vi "Game Engine.vi"(11 "Name(\"\" to use uuid)":string="Game Engine") -> ()   [LabVIEW 2020]
uses:
  <userlib>/_NEVSTOP/Communicable State Machine(CSM)/_Support/Priority Queue/Priority Queue.lvclass/Priority Queue.ctl
  <userlib>/_NEVSTOP/Communicable State Machine(CSM)/_Polymophic/Build Register Status Message.vi
  8ce7bf74-21e7-4c02-a855-96395cb58a13.vi
  7715e510-30ac-4bfd-a476-9bbe489e10a7.vi
  48a5b973-feea-438c-9c26-a61a5607df39.vi
  <userlib>/_NEVSTOP/Communicable State Machine(CSM)/_Polymophic/Build No-Reply Asynchronous Message with Arguments.vi
  b6e4d1e1-b2b0-4aba-8ccc-cc7579037c6e.vi
  bd3d81b0-0b8a-4f04-8495-35937f111f97.vi
  f528fd67-b2af-4e3f-99d6-bbe3ff85b99e.vi
  <vilib>/numeric/Random Number (Range) U64.vi
  b905f506-a76b-4f68-b7bf-6c6363b0f74c.vi
  0e950cba-ded0-4f4e-8f3c-d05bba4cd89c.vi
  <userlib>/_NEVSTOP/Communicable State Machine(CSM)/_Support/Process/CSMP-Async Call.vi
  <userlib>/_NEVSTOP/Communicable State Machine(CSM)/_Support/GlobalEvent/GEvt-Generate Status Log.vi
  <userlib>/_NEVSTOP/Communicable State Machine(CSM)/_Support/Process/CSMP-Broadcast.vi
  <userlib>/_NEVSTOP/Communicable State Machine(CSM)/_Support/GlobalEvent/GEvt-Generate Interrupt Log.vi
  <userlib>/_NEVSTOP/Communicable State Machine(CSM)/_Support/GlobalEvent/GEvt-Generate Register Log.vi
  <userlib>/_NEVSTOP/Communicable State Machine(CSM)/_Support/Process/CSMP-Register Status.vi
  <userlib>/_NEVSTOP/Communicable State Machine(CSM)/_Support/GlobalEvent/GEvt-Generate Unregister Log.vi
  <userlib>/_NEVSTOP/Communicable State Machine(CSM)/_Support/Process/CSMP-Unregister Status.vi
  <userlib>/_NEVSTOP/Communicable State Machine(CSM)/_Support/Process/CSMP-Sync Call.vi
  <userlib>/_NEVSTOP/Communicable State Machine(CSM)/_Support/CSMQ/_CSMObj-Unlock.vi
  <userlib>/_NEVSTOP/Communicable State Machine(CSM)/_Support/Process/CSMP-PostPostMsg.vi
  <userlib>/_NEVSTOP/Communicable State Machine(CSM)/_Support/Process/CSMP-PostSendMsg.vi
  <userlib>/_NEVSTOP/Communicable State Machine(CSM)/_Support/CSMQ/_CSMObj-Lock State.vi
  <userlib>/_NEVSTOP/Communicable State Machine(CSM)/_Support/Common/Splite Reason String Part.vi
  <userlib>/_NEVSTOP/Communicable State Machine(CSM)/_Support/Common/Trim Single line Text.vi
  <userlib>/_NEVSTOP/Communicable State Machine(CSM)/_Support/CSMQ/_CSMOFGV Release.vi
  <userlib>/_NEVSTOP/Communicable State Machine(CSM)/_Support/Common/Remove Comments from Line.vi
  <userlib>/_NEVSTOP/Communicable State Machine(CSM)/_Support/Common/Splite Single-line Message.vi
  <userlib>/_NEVSTOP/Communicable State Machine(CSM)/_Support/Common/Parse Next Single-line State.vi
  <userlib>/_NEVSTOP/Communicable State Machine(CSM)/_Support/CSMQ/_CSMOFGV Dequeue.vi
  <userlib>/_NEVSTOP/Communicable State Machine(CSM)/_Support/CSMQ/_CSMObj-Log Error if in a Remote Session.vi
  <userlib>/_NEVSTOP/Communicable State Machine(CSM)/_Support/GlobalEvent/GEvt-Generate State Change Log.vi
  <userlib>/_NEVSTOP/Communicable State Machine(CSM)/_Support/GlobalEvent/GEvt-Generate Remaining States Log.vi
  <userlib>/_NEVSTOP/Communicable State Machine(CSM)/_Support/GlobalEvent/GEvt-Generate Module Destroyed Log.vi
  <userlib>/_NEVSTOP/Communicable State Machine(CSM)/_Support/GlobalEvent/GEvt-Generate Complete Log.vi
  <userlib>/_NEVSTOP/Communicable State Machine(CSM)/_Support/GlobalEvent/GEvt-Generate Module Created Log.vi
  <userlib>/_NEVSTOP/Communicable State Machine(CSM)/_Support/GlobalEvent/Cache-GEvt Filter Object.vi
  <userlib>/_NEVSTOP/Communicable State Machine(CSM)/_Support/Common/Format Timestamp.vi
  <userlib>/_NEVSTOP/Communicable State Machine(CSM)/AdvanceAPI/CSM - Revert Arguments-Safe String.vi
  <userlib>/_NEVSTOP/Communicable State Machine(CSM)/AdvanceAPI/CSM - Make String Arguments Safe.vi
  <userlib>/_NEVSTOP/Communicable State Machine(CSM)/AdvanceAPI/CSM - Break Down Multiple States String.vi
  <userlib>/_NEVSTOP/Communicable State Machine(CSM)/AdvanceAPI/CSM - Compact Multiple States.vi
  <userlib>/_NEVSTOP/Communicable State Machine(CSM)/Utility/Trim Both Whitespace.vi
  <vilib>/numeric/sub_Random U32.vi
  <userlib>/_NEVSTOP/Communicable State Machine(CSM)/_Support/CSMQ/_CSMObj-Message Check.vi
  <userlib>/_NEVSTOP/Communicable State Machine(CSM)/_Support/CSMQ/_CSMObj-Enqueue Cross-Module Message.vi
  <userlib>/_NEVSTOP/Communicable State Machine(CSM)/_Support/CSMQ/_CSMOFGV Get.vi
  <userlib>/_NEVSTOP/Communicable State Machine(CSM)/_Support/GlobalEvent/GEvt-Generate with Rule Check.vi
  <userlib>/_NEVSTOP/Communicable State Machine(CSM)/_Support/FGV-BroadcastRegistry/Cache-Broadcast Registry Search Result.vi
  <userlib>/_NEVSTOP/Communicable State Machine(CSM)/AdvanceAPI/CSM - Register Status Change.vi
  <userlib>/_NEVSTOP/Communicable State Machine(CSM)/AdvanceAPI/CSM - Unregister Status Change.vi
  <userlib>/_NEVSTOP/Communicable State Machine(CSM)/_Support/Common/Hex Str to U8 Data.vi
  <userlib>/_NEVSTOP/Communicable State Machine(CSM)/_Support/Common/Concatenate State with Arguments.vi
  <userlib>/_NEVSTOP/Communicable State Machine(CSM)/_Support/Common/U8 Data to Hex Str.vi
  <userlib>/_NEVSTOP/Communicable State Machine(CSM)/_Support/Priority Queue/Dequeue Element.vi
  <userlib>/_NEVSTOP/Communicable State Machine(CSM)/AdvanceAPI/CSM - Keywords.vi
  <userlib>/_NEVSTOP/Communicable State Machine(CSM)/_Support/Priority Queue/Enqueue Element.vi
  <userlib>/_NEVSTOP/Communicable State Machine(CSM)/_Support/GlobalEvent/LogFilter/Filter Check.vi
  <userlib>/_NEVSTOP/Communicable State Machine(CSM)/_Support/GlobalEvent/FGV-GlobalEventRef.vi
  <userlib>/_NEVSTOP/Communicable State Machine(CSM)/_Support/GlobalEvent/global-GEvnt Filter Change Flag.vi
  <userlib>/_NEVSTOP/Communicable State Machine(CSM)/FGV-GEvt Filter Obj.vi
  <userlib>/_NEVSTOP/Communicable State Machine(CSM)/_Support/CSMQ/_CSMOFGV Obtain.vi
  <userlib>/_NEVSTOP/Communicable State Machine(CSM)/_Support/GlobalEvent/LogFilter/CheckVIs/Group Check - CSM.vi
  <userlib>/_NEVSTOP/Communicable State Machine(CSM)/_Support/GlobalEvent/LogFilter/CheckVIs/Group Check - LogType.vi
  <userlib>/_NEVSTOP/Communicable State Machine(CSM)/_Support/GlobalEvent/LogFilter/CheckVIs/Group Check - State.vi
  <userlib>/_NEVSTOP/Communicable State Machine(CSM)/_Support/GlobalEvent/LogFilter/CheckVIs/CSM Check - LogType.vi
  <userlib>/_NEVSTOP/Communicable State Machine(CSM)/_Support/GlobalEvent/LogFilter/CheckVIs/CSM Check - State.vi
  <userlib>/_NEVSTOP/Communicable State Machine(CSM)/_Support/GlobalEvent/LogFilter/CheckVIs/CSM Check - StateType.vi
  <userlib>/_NEVSTOP/Communicable State Machine(CSM)/_Support/GlobalEvent/LogFilter/CheckVIs/Group Check - StateType.vi
  <userlib>/_NEVSTOP/Communicable State Machine(CSM)/_Support/CSMQ/_CSMOFGV.vi
  <userlib>/_NEVSTOP/Communicable State Machine(CSM)/_Support/Error/CSM Not Allowed Message.vi
  <userlib>/_NEVSTOP/Communicable State Machine(CSM)/_Support/GlobalEvent/FGV-StatusChangeEventRef.vi
  <userlib>/_NEVSTOP/Communicable State Machine(CSM)/_Support/FGV-BroadcastRegistry/global-CSMQ FGV Change Flag.vi
  <userlib>/_NEVSTOP/Communicable State Machine(CSM)/_Support/FGV-BroadcastRegistry/global-Broadcast Cache Change Flag.vi
  <userlib>/_NEVSTOP/Communicable State Machine(CSM)/_Support/BroadcastRegistry/HelperVI/Broadcast Item Key.vi
  <userlib>/_NEVSTOP/Communicable State Machine(CSM)/_Support/FGV-BroadcastRegistry/FGV-BroadcastRegistry.vi
  <userlib>/_NEVSTOP/Communicable State Machine(CSM)/_Support/Message/Parse Register Message.vi
  <userlib>/_NEVSTOP/Communicable State Machine(CSM)/_Support/Message/Parse Unregister Message.vi
  <userlib>/_NEVSTOP/Communicable State Machine(CSM)/addons/API-String-Arugments-Support/_Support/Convert API String Arguments to Data(variant).vi
  <userlib>/_NEVSTOP/Communicable State Machine(CSM)/addons/API-String-Arugments-Support/_Support/Data To API String Arguments.vi
  <userlib>/_NEVSTOP/Communicable State Machine(CSM)/_Support/Message/Parse State with Arguments String.vi
  <userlib>/_NEVSTOP/Communicable State Machine(CSM)/Communicable State Machine.lvlib
panel:
  out "Error Occurred":errorcluster
  out "State History":string
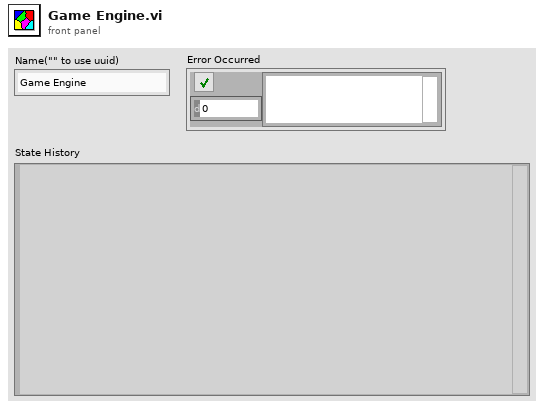
[diagram p1: front panel]
types:
  T1 = enum32{"Invalid", "Standard", "Closed", "Hidden", "Minimized", "Maximized"}
  T2 = enum32{"invalid app kind", "Development System", "Run Time System", "Student Edition", "Embedded LabVIEW", "Evaluation", "Custom"}
  T3 = typedef "Communicable State Machine.lvlib/_CSM_Response Source Message.ctl" = cluster{"‘State":string, "’Arguments":string, "’Error":errorcluster}
  T4 = cluster{"Current VI Reference":refnum<vi>, "Close Panel on Exit?":bool}
  T5 = cluster{"Core":cluster{"Current VI Reference":refnum<vi>, "Close Panel on Exit?":bool}, "Your Boolean data":bool, "current":timestamp, "timeseq":cluster{"SEQ":i32[], "time":i32}, "score":i32, "TAPSEQ":i32[], "elapsed":dbl, "load":dbl}
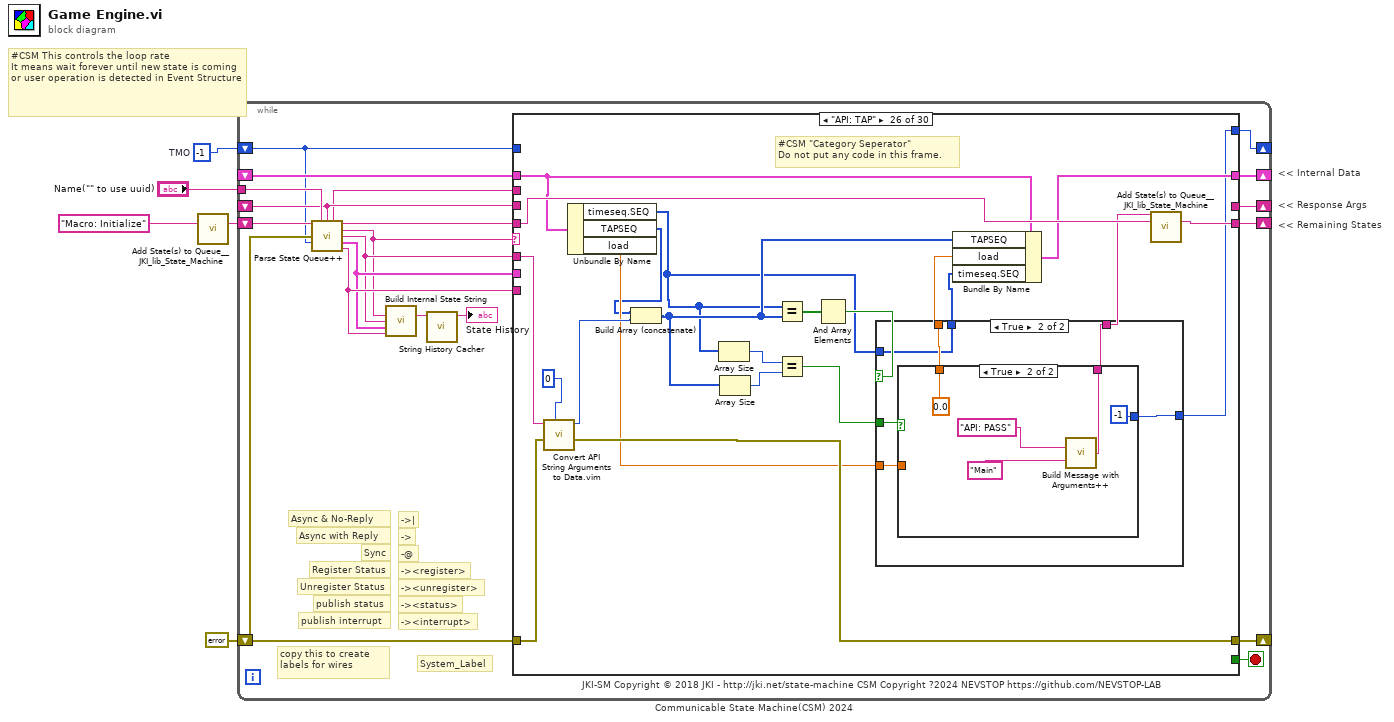
[diagram p0: block diagram]
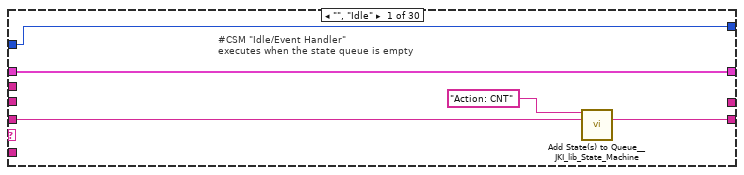
[diagram p2: hidden frame]
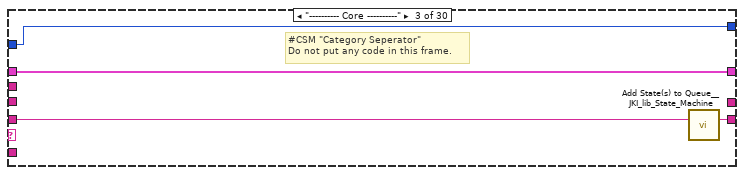
[diagram p4: hidden frame]
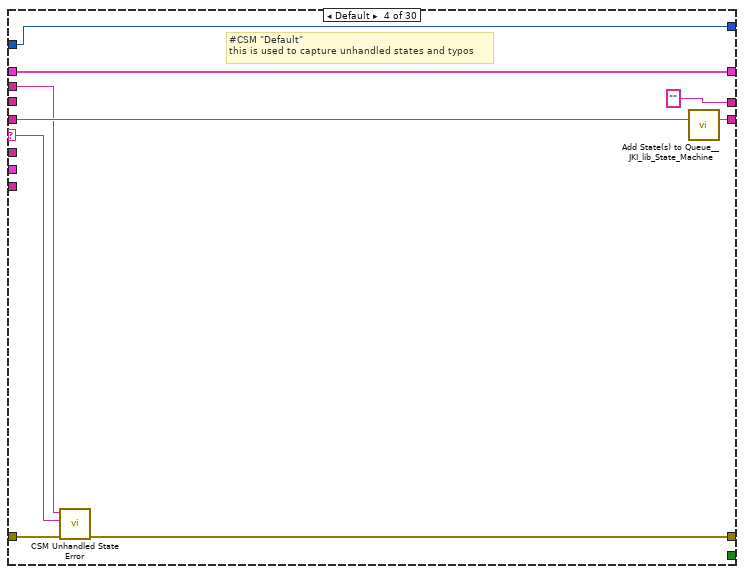
[diagram p5: hidden frame]
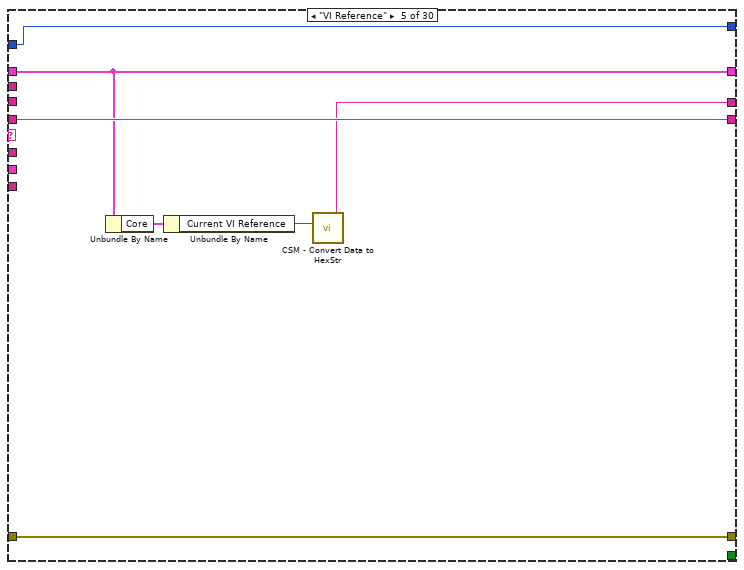
[diagram p6: hidden frame]
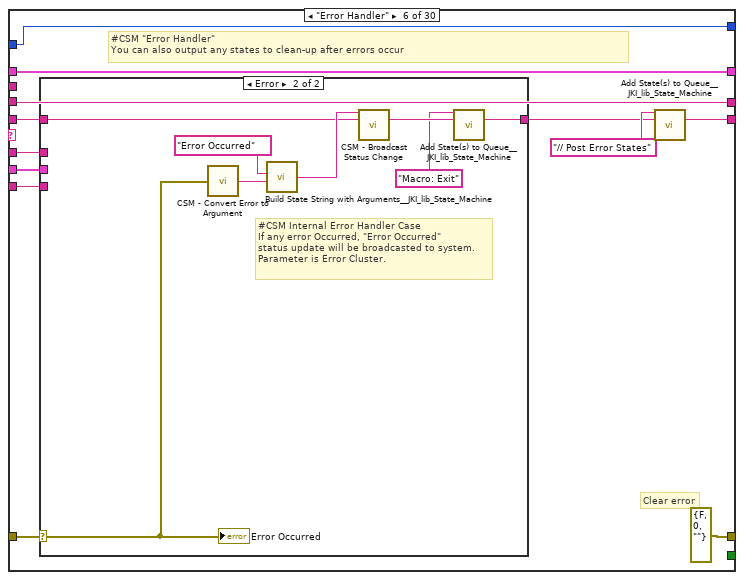
[diagram p7: hidden frame]
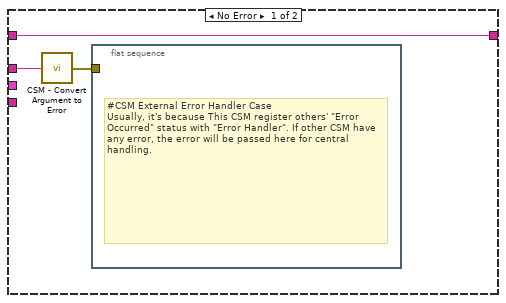
[diagram p8: hidden frame]
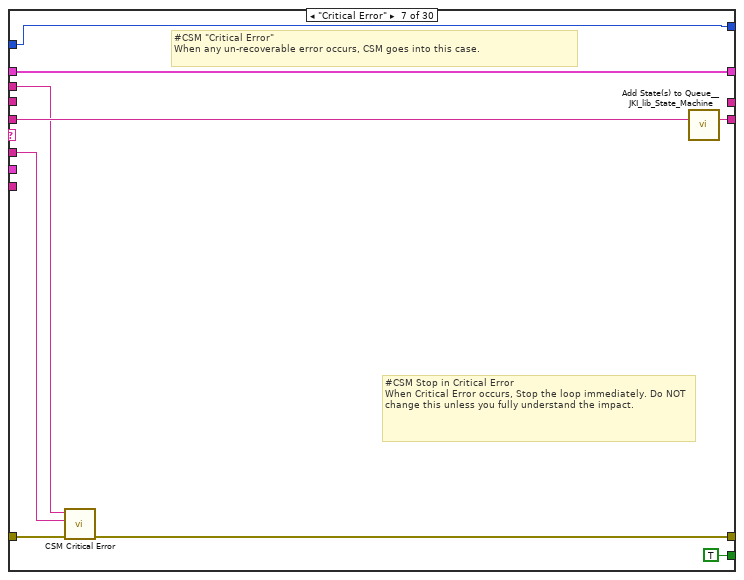
[diagram p9: hidden frame]
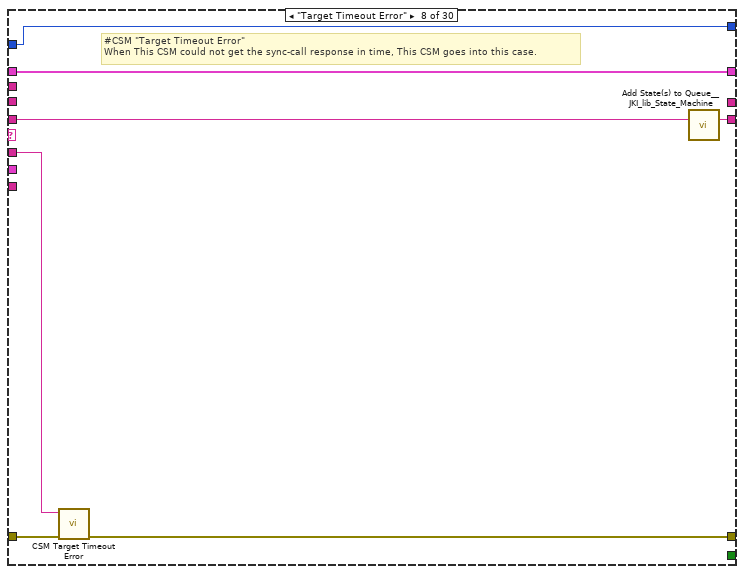
[diagram p10: hidden frame]
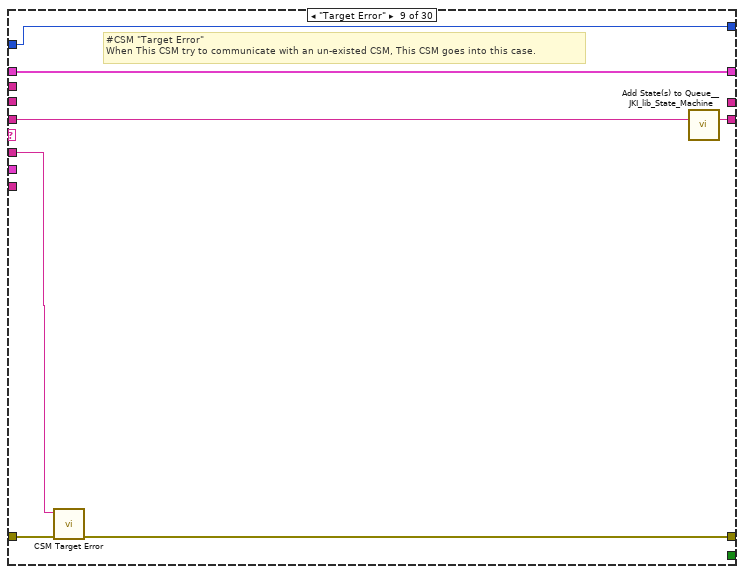
[diagram p11: hidden frame]
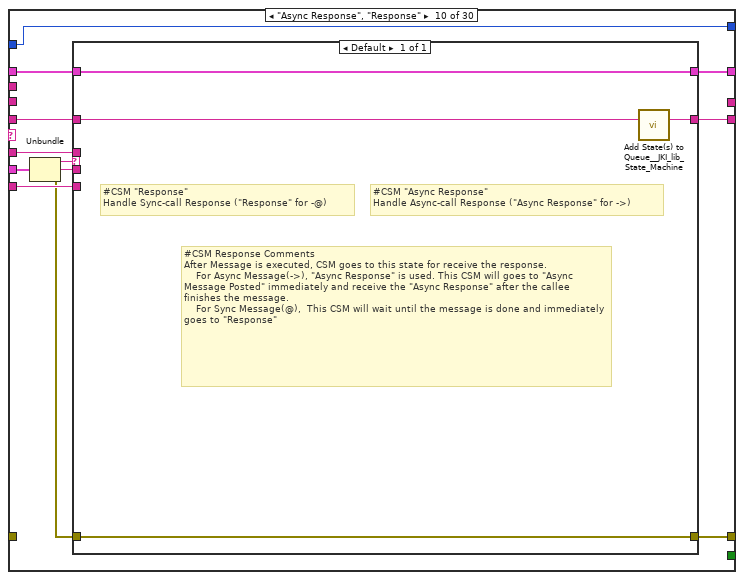
[diagram p12: hidden frame]
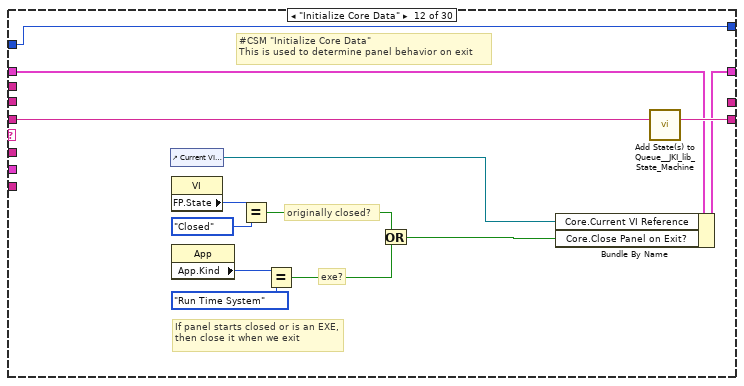
[diagram p14: hidden frame]
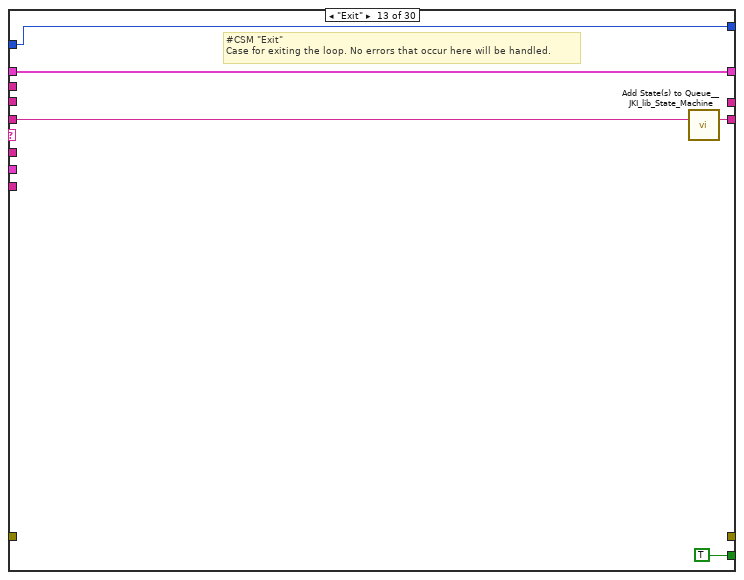
[diagram p15: hidden frame]
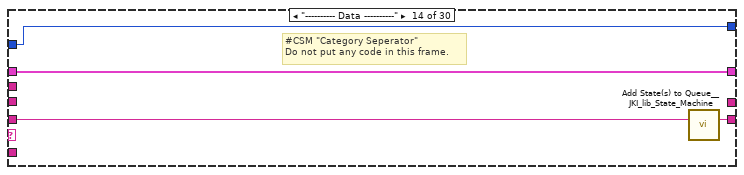
[diagram p16: hidden frame]
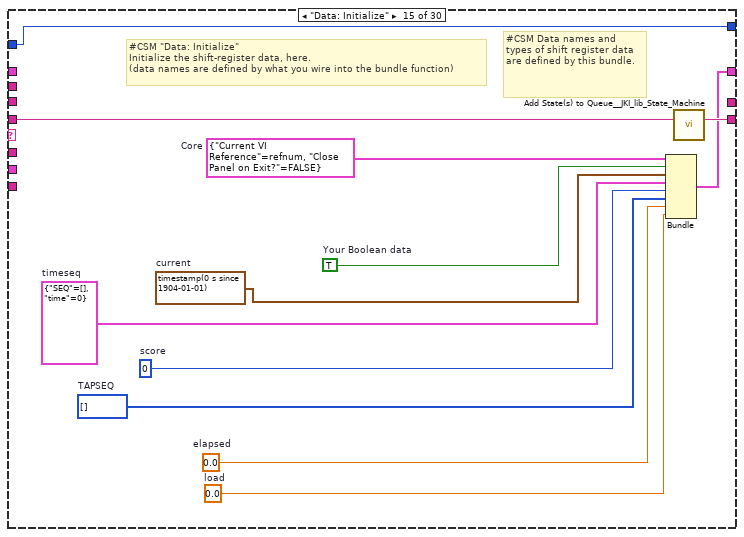
[diagram p17: hidden frame]
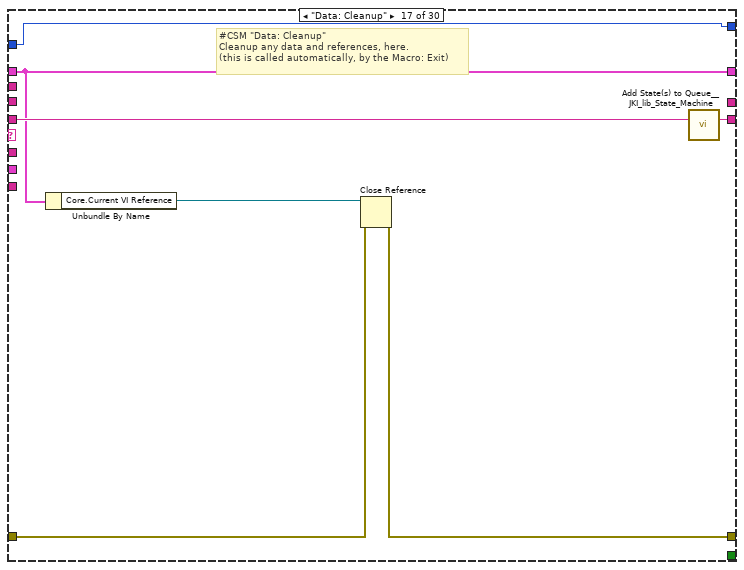
[diagram p19: hidden frame]
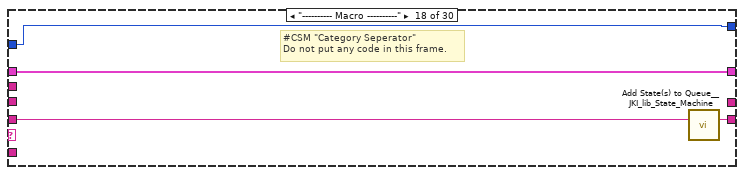
[diagram p20: hidden frame]
diagram:
  w1 = -1  # TMO
  # "#CSM This controls the loop rate\nIt means wait forever until new state is coming or user operation is detected in Event Structure"
  # "<< Internal Data"
  # "<< Response Args"
  # "<< Remaining States"
  n1 = call <vilib>:"Add State(s) to Queue__JKI_lib_State_Machine.vi"("State(s) in (\"\")"="Macro: Initialize" ("Init State(\"Macro: Initialize\")")) -> ("States Out"=w3:string)  [unwired: 14 in]
  n2 = while "Communicable State Machine(CSM) 2024" {
    shift-right: [w20] -> _
    shift-left: _ -> [w19]
    shift-right: [w23] -> _
    shift-left: errorcluster {"status"=FALSE, "code"=0, "source"=""} ("error out") -> [w8]
    shift-right: [w22] -> _
    shift-left: w3 -> [w24]
    tunnel: "Name(\"\" to use uuid)" -> [w17]
    shift-right: [w18] -> _
    shift-left: _ -> [w10]
    shift-right: [w7] -> _
    shift-left: w1 -> [w6]
    stop <- w21 stop-if-true
    # "-><interrupt>"
    # "-><status>"
    # "-><unregister>"
    # "-><register>"
    # "-@"
    # "->"
    # "->|"
    # "publish interrupt"
    # "publish status"
    # "Unregister Status"
    # "Register Status"
    # "Sync"
    # "Async with Reply"
    # "Async & No-Reply"
    # "JKI-SM Copyright © 2018 JKI - http://jki.net/state-machine CSM Copyright ?2024 NEVSTOP https://github.com/NEVSTOP-LAB"
    # "copy this to create labels for wires"
    # "System_Label"
    n3 = call <userlib>:"Parse State Queue++.vi"("State Queue"=w24, "Name(\"\" to use uuid)"=w17, "Response Arguments"=w10, "Error In (no error)"=w8, "Dequeue Timeout(0ms)"=w6) -> ("Name Used"=w9:string, "Remaining States"=w25:string, "Current State"=w11:string, "Arguments"=w12:string, ">> Response Source Message >>"=w13:T3, ">> Source CSM >>"=w14:string)  [unwired: 5 in]
    n4 = call <userlib>:"Build Internal State String.vi"("State"=w11, "Arguments (\"\")"=w12, ">> Response Source Message >>"=w13, "Source (\"\")"=w14) -> ("State with Arguments"=w15:string)  [unwired: 11 in]
    n5 = call <userlib>:"String History Cacher.vi"("String"=w15) -> ("String Cache"=→"State History":string)  [unwired: 10 in]
    n6 = case shown="\"API: TAP\"" w11 {
      selector: w11 -> [_ _ _ w42 _ _ _ _ _ _ _ _ _ _ _ _ _ _ _ _ _ _ _ _ _ _ _ _ _ _]
      tunnel: w25 -> [w28 w33 w37 w46 w52 w59 w85 w92 w99 w110 w118 w131 w136 w140 w152 w155 w162 w166 w170 w188 w191 w200 w213 w231 w249 w267 w296 w305 w333 w348]
      tunnel: w12 -> [_ _ _ _ _ w58 w81 w89 w96 w104 _ _ _ _ _ _ _ _ _ _ _ w205 w211 _ w242 w265 _ _ _ _]
      tunnel: w19 -> [w30 w32 w35 w44 w51 w64 w83 w90 w97 w108 w117 w125 w134 w138 _ w154 w157 w164 w180 w186 w190 w195 w216 w221 w238 w261 w294 w311 w322 w345]
      tunnel: [_ _ _ w39 w53 errorcluster {"status"=FALSE, "code"=0, "source"=""} ("error out") w78 w87 w94 w111 _ _ _ _ _ _ w158 _ _ _ _ w198 w208 w222 w243 w257 _ w313 w319 _] -> w23
      tunnel: w8 -> [_ _ _ w40 w53 w62 w79 w88 w95 _ _ _ _ _ _ _ w159 _ _ _ _ w204 w210 w223 w241 w263 _ w298 w320 _]
      tunnel: [w29 w33 w36 w45 w52 w60 w84 w91 w98 w109 w118 w130 w135 w139 w151 w155 w161 w165 w181 w187 w191 w201 w214 w232 w250 w268 w295 w306 w334 w347] -> w22
      tunnel: [_ _ _ _ _ _ TRUE _ _ _ _ _ TRUE _ _ _ _ _ _ _ _ _ _ _ _ _ _ _ _ _] -> w21
      tunnel: [w30 w32 w35 w44 w51 w64 w83 w90 w97 w107 w117 w129 w134 w138 w150 w154 w157 w164 w180 w186 w190 w203 w215 w220 w236 w260 w294 w312 w321 w344] -> w20
      tunnel: w14 -> [_ _ _ _ _ w57 _ _ _ w105 _ _ _ _ _ _ _ _ _ _ _ _ _ _ _ _ _ _ _ _]
      tunnel: w13 -> [_ _ _ _ _ w56 _ _ _ w106 _ _ _ _ _ _ _ _ _ _ _ _ _ _ _ _ _ _ _ _]
      tunnel: [_ _ _ "" w48 w55 _ _ _ _ _ _ _ _ _ _ _ _ _ _ _ _ _ _ _ _ _ _ _ _] -> w18
      tunnel: w9 -> [_ _ _ w41 _ _ w80 _ _ _ _ _ _ _ _ _ _ _ w167 _ _ _ _ _ _ _ _ _ _ _]
      tunnel: w10 -> [_ _ _ _ _ w55 _ _ _ _ _ _ _ _ _ _ _ _ _ _ _ _ _ _ _ _ _ _ _ _]
      tunnel: [w27 w31 w34 w38 w47 w54 w77 w86 w93 w100 w116 w119 w132 w137 w145 w153 w156 w163 w175 w182 w189 w196 w212 -1 ("TMO") 100 ("TMO") w256 w293 w297 w323 -1 ("TMO")] -> w7
      tunnel: w6 -> [w27 w31 w34 w38 w47 w54 w77 w86 w93 w100 w116 w119 w132 w137 w145 w153 w156 w163 w175 w182 w189 w196 w212 _ _ _ w293 w297 _ _]
      frame "", "Idle" {
        # "#CSM \"Idle/Event Handler\"\nexecutes when the state queue is empty"
        n7 = call <vilib>:"Add State(s) to Queue__JKI_lib_State_Machine.vi"("State(s) in Front (\"\")"="Action: CNT" ("State(s) in Front (\"\")"), "State(s) in (\"\")"=w28) -> ("States Out"=w29:string)  [unwired: 13 in]
      }
      frame "CSM Documentation" {
        # "#CSM Documentation"
        # "#CSM State Syntax\n\n// Comment line, all text to the right of “//” will be ignored\n// Local Message Example\nDoSth: DoA >> Arguments\n\n// Sync Call Example\nAPI: xxxx >> Arguments -@ TargetModule\n\n// Async Call Example\nAPI: xxxx >> Arguments -> TargetModule\n\n// Async Call without Reply Example\nAPI: xxxx >> Arguments ->| TargetModule\n\n// Broadcast normal status:\nStatus >> StatusArguments  -><status>\n\n// Broadcast Interrupt status:\nInterrupt >> StatusArguments  -><interrupt>\n\n// Register Source Module's status to Handler Module\nStatus@Source Module >> Handler Module@Handler Module -><register>\n\n// Unegister Source Module's status\nStatus@Source Module >> Handler Module -><unregister>"
        # "#CSM README FIRST\n\nCommunicable State Machine(CSM) is a LabVIEW application framework that builds upon JKI State Machine(JKISM). It follows the pattern of JKISM and extends the keywords to describe message communication between modules, including concepts such as Sync-Message, Async-Message, Subscription/Unsubscription of status - essential elements for creating reusable code modules. For more information, please visit the CSM wiki: https://nevstop-lab.github.io/CSM-Wiki/\n\nFor instructions on JKI State Machine, visit: \n    http://jki.net/state-machine/\nFor information about CSM, visit: \n    https://github.com/NEVSTOP-LAB"
        # "#CSM \"Documentation\"\nCase for holding CSM Documenation"
      }
      frame "---------- Core ----------" {
        # "#CSM \"Category Seperator\"\nDo not put any code in this frame."
        n8 = call <vilib>:"Add State(s) to Queue__JKI_lib_State_Machine.vi"("State(s) in (\"\")"=w37) -> ("States Out"=w36:string)  [unwired: 14 in]
      }
      frame Default {
        # "#CSM \"Default\"\nthis is used to capture unhandled states and typos"
        n9 = call <userlib>:"CSM Unhandled State Error.vi"("error in (no error)"=w40, "Current State"=w42, "CSM Name"=w41) -> ("error out"=w39:errorcluster)  [unwired: 8 in]
        n10 = call <vilib>:"Add State(s) to Queue__JKI_lib_State_Machine.vi"("State(s) in (\"\")"=w46) -> ("States Out"=w45:string)  [unwired: 14 in]
      }
      frame "VI Reference" {
        n11 = Unbundle By Name(w51) -> ("Core"=w50:T4)
        n12 = Unbundle By Name(w50) -> ("Current VI Reference"=w49:refnum<vi>)
        n13 = call <userlib>:"CSM - Convert Data to HexStr.vi"("Variant"=w49) -> ("HEX String (0-9,A-F)"=w48:string)  [unwired: 8 in]
      }
      frame "Error Handler" {
        # "#CSM \"Error Handler\"\nYou can also output any states to clean-up after errors occur"
        # "Clear error"
        n14 = case shown="Error" w62 {
          selector: w62 -> [_ w72]
          tunnel: [w68 w71] -> w61
          tunnel: w59 -> [w68 w73]
          tunnel: w58 -> [w67 _]
          tunnel: w57 -> [_ _]
          tunnel: w56 -> [_ _]
          frame No Error {
            n15 = call <userlib>:"CSM - Convert Argument to Error.vi"("Argument"=w67) -> ("error"=w66:errorcluster)  [unwired: 4 in]
            n16 = flat-sequence {
              tunnel: w66 -> [_]
              frame #0 {
                # "#CSM External Error Handler Case\nUsually, it's because This CSM register others' \"Error Occurred\" status with \"Error Handler\". If other CSM have any error, the error will be passed here for central handling."
              }
            }
          }
          frame Error {
            # "#CSM Internal Error Handler Case \nIf any error Occurred, \"Error Occurred\" \nstatus update will be broadcasted to system.\nParameter is Error Cluster."
            n17 = call <userlib>:"CSM - Convert Error to Argument.vi"("error in (no error)"=w72) -> ("Arguments"=w75:string)  [unwired: 4 in]
            n18 = call <vilib>:"Build State String with Arguments__JKI_lib_State_Machine.vi"("Arguments (\"\")"=w75, "State"="Error Occurred" ("Status with Arguments")) -> ("State with Arguments"=w74:string)  [unwired: 4 in]
            n19 = call <userlib>:"CSM - Broadcast Status Change.vi"("Status with Arguments"=w74, "State Queue"=w73) -> ("Remaining States"=w70:string)  [unwired: 13 in]
            n20 = call <vilib>:"Add State(s) to Queue__JKI_lib_State_Machine.vi"("State(s) in Front (\"\")"="Macro: Exit" ("State(s) in Front (\"\")"), "State(s) in (\"\")"=w70) -> ("States Out"=w71:string)  [unwired: 13 in]
            "Error Occurred" <- w72
          }
        }
        n21 = call <vilib>:"Add State(s) to Queue__JKI_lib_State_Machine.vi"("State(s) in Front (\"\")"="// Post Error States", "State(s) in (\"\")"=w61) -> ("States Out"=w60:string)  [unwired: 13 in]
      }
      frame "Critical Error" {
        # "#CSM \"Critical Error\"\nWhen any un-recoverable error occurs, CSM goes into this case."
        # "#CSM Stop in Critical Error\nWhen Critical Error occurs, Stop the loop immediately. Do NOT change this unless you fully understand the impact."
        n22 = call <userlib>:"CSM Critical Error.vi"("error in (no error)"=w79, "Arugments(as Reason)"=w81, "CSM Name"=w80) -> ("error out"=w78:errorcluster)  [unwired: 8 in]
        n23 = call <vilib>:"Add State(s) to Queue__JKI_lib_State_Machine.vi"("State(s) in (\"\")"=w85) -> ("States Out"=w84:string)  [unwired: 14 in]
      }
      frame "Target Timeout Error" {
        # "#CSM \"Target Timeout Error\"\nWhen This CSM could not get the sync-call response in time, This CSM goes into this case."
        n24 = call <userlib>:"CSM Target Timeout Error.vi"("error in (no error)"=w88, "Arguments(as CSM Name)"=w89) -> ("error out"=w87:errorcluster)  [unwired: 9 in]
        n25 = call <vilib>:"Add State(s) to Queue__JKI_lib_State_Machine.vi"("State(s) in (\"\")"=w92) -> ("States Out"=w91:string)  [unwired: 14 in]
      }
      frame "Target Error" {
        # "#CSM \"Target Error\"\nWhen This CSM try to communicate with an un-existed CSM, This CSM goes into this case."
        n26 = call <userlib>:"CSM Target Error.vi"("error in (no error)"=w95, "Arguments(as CSM Name)"=w96) -> ("error out"=w94:errorcluster)  [unwired: 9 in]
        n27 = call <vilib>:"Add State(s) to Queue__JKI_lib_State_Machine.vi"("State(s) in (\"\")"=w99) -> ("States Out"=w98:string)  [unwired: 14 in]
      }
      frame "Async Response", "Response" {
        n28 = Unbundle(w106) -> ("‘State"=w103:string, "’Arguments"=w102:string, "’Error"=w101:errorcluster)
        n29 = case shown="Default" w103 {
          tunnel: [w112] -> w109
          tunnel: w110 -> [w113]
          tunnel: [w115] -> w107
          tunnel: w108 -> [w115]
          tunnel: [w114] -> w111
          tunnel: w101 -> [w114]
          tunnel: w105 -> [_]
          tunnel: w104 -> [_]
          tunnel: w102 -> [_]
          frame Default {
            # "#CSM \"Async Response\"\nHandle Async-call Response (\"Async Response\" for ->)"
            # "#CSM \"Response\"\nHandle Sync-call Response (\"Response\" for -@)"
            # "#CSM Response Comments\nAfter Message is executed, CSM goes to this state for receive the response.\n    For Async Message(->), \"Async Response\" is used. This CSM will goes to \"Async Message Posted\" immediately and receive the \"Async Response\" after the callee finishes the message.\n    For Sync Message(@),  This CSM will wait until the message is done and immediately goes to \"Response\""
            n30 = call <vilib>:"Add State(s) to Queue__JKI_lib_State_Machine.vi"("State(s) in (\"\")"=w113) -> ("States Out"=w112:string)  [unwired: 14 in]
          }
        }
      }
      frame "Async Message Posted" {
        # "#CSM \"Async Message Posted\"\nAfter Async Message is posted (-> or ->| ), CSM goes to this state for post-action.\nYou can use Argument - State to tell which Async Message is called."
      }
      frame "Initialize Core Data" {
        # "#CSM \"Initialize Core Data\"\nThis is used to determine panel behavior on exit"
        # "originally closed?"
        # "exe?"
        # "If panel starts closed or is an EXE, then close it when we exit"
        n31 = control-ref of="Current VI Reference"() -> (w123:refnum<vi>)
        n32 = property class="VI"() -> ("FP.State"=w122:T1)  [unwired: 2 in, 2 out]
        n33 = property class="App"() -> ("App.Kind"=w128:T2)  [unwired: 2 in, 2 out]
        n34 = Equal?(x=w122, y=T1."Closed" ("Front Panel Window:State")) -> (x = y?=w120:bool)
        n35 = Equal?(x=w128, y=T2."Run Time System" ("Application:Kind")) -> (x = y?=w126:bool)
        n36 = Or(x=w120, y=w126) -> (x .or. y?=w124:bool)
        n37 = Bundle By Name(cluster=w125, "Core.Current VI Reference"=w123, "Core.Close Panel on Exit?"=w124) -> (w129:T5)
        n38 = call <vilib>:"Add State(s) to Queue__JKI_lib_State_Machine.vi"("State(s) in (\"\")"=w131) -> ("States Out"=w130:string)  [unwired: 14 in]
      }
      frame "Exit" {
        # "#CSM \"Exit\"\nCase for exiting the loop. No errors that occur here will be handled."
        n39 = call <vilib>:"Add State(s) to Queue__JKI_lib_State_Machine.vi"("State(s) in (\"\")"=w136) -> ("States Out"=w135:string)  [unwired: 14 in]
      }
      frame "---------- Data ----------" {
        # "#CSM \"Category Seperator\"\nDo not put any code in this frame."
        n40 = call <vilib>:"Add State(s) to Queue__JKI_lib_State_Machine.vi"("State(s) in (\"\")"=w140) -> ("States Out"=w139:string)  [unwired: 14 in]
      }
      frame "Data: Initialize" {
        w141 = 0.0  # load
        w142 = 0.0  # elapsed
        w143 = cluster{"SEQ":i32[], "time":i32} {"SEQ"=[], "time"=0}  # timeseq
        w144 = timestamp(0 s since 1904-01-01)  # current
        w146 = i32[] []  # TAPSEQ
        w147 = 0  # score
        w148 = T4 {"Current VI Reference"=refnum, "Close Panel on Exit?"=FALSE}  # Core
        w149 = TRUE  # Your Boolean data
        # "#CSM \"Data: Initialize\"\nInitialize the shift-register data, here.\n(data names are defined by what you wire into the bundle function)"
        # "#CSM Data names and types of shift register data are defined by this bundle."
        n41 = Bundle("Core"=w148, "Your Boolean data"=w149, "current"=w144, "timeseq"=w143, "score"=w147, "TAPSEQ"=w146, "elapsed"=w142, "load"=w141) -> (w150:T5)  [unwired: 1 in]
        n42 = call <vilib>:"Add State(s) to Queue__JKI_lib_State_Machine.vi"("State(s) in (\"\")"=w152) -> ("States Out"=w151:string)  [unwired: 14 in]
      }
      frame "Data: Update Indicators" {
      }
      frame "Data: Cleanup" {
        # "#CSM \"Data: Cleanup\"\nCleanup any data and references, here.\n(this is called automatically, by the Macro: Exit)"
        n43 = Unbundle By Name(w157) -> ("Core.Current VI Reference"=w160:refnum<vi>)
        n44 = Close Reference(reference=w160, error in (no error)=w159) -> (error out=w158:errorcluster)
        n45 = call <vilib>:"Add State(s) to Queue__JKI_lib_State_Machine.vi"("State(s) in (\"\")"=w162) -> ("States Out"=w161:string)  [unwired: 14 in]
      }
      frame "---------- Macro ----------" {
        # "#CSM \"Category Seperator\"\nDo not put any code in this frame."
        n46 = call <vilib>:"Add State(s) to Queue__JKI_lib_State_Machine.vi"("State(s) in (\"\")"=w166) -> ("States Out"=w165:string)  [unwired: 14 in]
      }
      frame "Macro: Initialize" {
        # "#CSM \"Macro: Initialize\"\nInitialization Macro (This is called once, when the VI starts)"
        n47 = call-poly <userlib>:"Build Message with Arguments++.vi"("CSM Name"=w167, "Source CSM Name (* as Default)"="*", "Status"="EXIT", "Response Message (if \"\", same as Source Message)"="Macro: Exit" ("Response Message (if \"\", same as Source Message)")) -> ("State with Arguments"=w169:string)  [unwired: 11 in]
        n48 = call-poly <userlib>:"Build Message with Arguments++.vi"("CSM Name"=w167, "Source CSM Name (* as Default)"="*", "Status"="GAMEEXIT", "Response Message (if \"\", same as Source Message)"="Action: EXIT" ("Response Message (if \"\", same as Source Message)")) -> ("State with Arguments"=w168:string)  [unwired: 11 in]
        n49 = call <vilib>:"Add State(s) to Queue__jki_lib_state_machine.vi"("State(s) in Front (\"\")"=w169, "State(s) in (\"\")"=w170, "State(s) at Back (\"\")"=w168) -> ("States Out"=w171:string)  [unwired: 12 in]
        n50 = call <vilib>:"Add State(s) to Queue__JKI_lib_State_Machine.vi"("State(s) in Front (\"\")"="Data: Initialize\nInitialize Core Data\nData: Update Indicators", "State(s) in (\"\")"=w171) -> ("States Out"=w181:string)  [unwired: 13 in]
      }
      frame "Macro: Exit" {
        # "#CSM \"Macro: Exit\"\nExit Macro (This is called once, when the VI exits)"
        n51 = call <vilib>:"Add State(s) to Queue__JKI_lib_State_Machine.vi"("State(s) in Front (\"\")"="//Exit Sub-Modules ", "State(s) at Back (\"\")"="Data: Cleanup\nExit") -> ("States Out"=w184:string)  [unwired: 13 in]
        n52 = call <vilib>:"Add State(s) to Queue__JKI_lib_State_Machine.vi"("State(s) in Front (\"\")"=w184, "State(s) in (\"\")"=w188) -> ("States Out"=w187:string)  [unwired: 13 in]
      }
      frame "---------- API ----------" {
        # "#CSM \"Category Seperator\"\nDo not put any code in this frame."
      }
      frame "API: SEQ" {
        # "#CSM API Example\nCopy/Rename this case for your own API"
        n53 = Unbundle By Name(w195) -> ("timeseq"=w194:cluster{"SEQ":i32[], "time":i32})
        n54 = call "Convert API String Arguments to Data.vim"("Type"=w194, "error in (no error)"=w204, "String"=w205) -> ("error"=w198:errorcluster, "Data"=w192:cluster{"SEQ":i32[], "time":i32})  [unwired: 5 in]
        n55 = Unbundle By Name(w192) -> ("SEQ"=w193:i32[])
        n56 = Array Size(array=w193) -> (size(s)=w199:i32)
        n57 = Bundle By Name(cluster=w195, "TAPSEQ"=i32[] [], "score"=w199, "timeseq"=w192) -> (w203:T5)
        n58 = call <vilib>:"Add State(s) to Queue__JKI_lib_State_Machine.vi"("State(s) in Front (\"\")"="Action: SEQ" ("State(s) in Front (\"\")"), "State(s) in (\"\")"=w200) -> ("States Out"=w201:string)  [unwired: 13 in]
      }
      frame "API: CNT" {
        # "#CSM API Example\nCopy/Rename this case for your own API"
        n59 = Get Date/Time In Seconds() -> (seconds since 1Jan1904=w206:timestamp)
        n60 = call "Convert API String Arguments to Data.vim"("Type"=w206, "error in (no error)"=w210, "String"=w211) -> ("error"=w208:errorcluster, "Data"=w209:timestamp)  [unwired: 5 in]
        n61 = Bundle By Name(cluster=w216, "current"=w209) -> (w215:T5)
        n62 = call <vilib>:"Add State(s) to Queue__JKI_lib_State_Machine.vi"("State(s) in Front (\"\")"="Action: CNT" ("State(s) in Front (\"\")"), "State(s) in (\"\")"=w213) -> ("States Out"=w214:string)  [unwired: 13 in]
      }
      frame "API: PAUSE" {
        # "#CSM API Example\nCopy/Rename this case for your own API"
        n63 = Unbundle By Name(w221) -> ("current"=w225:timestamp, "load"=w218:dbl)
        n64 = Get Date/Time In Seconds() -> (seconds since 1Jan1904=w226:timestamp)
        n65 = Subtract(x=w226, y=w225) -> (x-y=w219:dbl)
        n66 = Add(x=w219, y=w218) -> (x+y=w217:dbl)
        n67 = Bundle By Name(cluster=w221, "load"=w217) -> (w220:T5)
        n68 = call "Convert Data To API String Arguments.vim"("error in (no error)"=w223, "data"=w217) -> ("error out"=w222:errorcluster, "String"=w229:string)  [unwired: 6 in]
        n69 = call-poly <userlib>:"Build Message with Arguments++.vi"("State with Arguments"="API: show", "Arguments (\"\")"=w229, "Target Module (\"\")"="Main" ("Target Module (\"\")")) -> ("State with Arguments out"=w227:string)  [unwired: 12 in]
        n70 = call <vilib>:"Add State(s) to Queue__JKI_lib_State_Machine.vi"("State(s) in Front (\"\")"=w227, "State(s) in (\"\")"=w231) -> ("States Out"=w232:string)  [unwired: 13 in]
      }
      frame "API: RESUME" {
        # "#CSM API Example\nCopy/Rename this case for your own API"
        n71 = Get Date/Time In Seconds() -> (seconds since 1Jan1904=w239:timestamp)
        n72 = call "Convert API String Arguments to Data.vim"("Type"=w239, "error in (no error)"=w241, "String"=w242) -> ("error"=w240:errorcluster, "Data"=w237:timestamp)  [unwired: 5 in]
        n73 = Bundle By Name(cluster=w238, "current"=w237) -> (w236:T5)
        n74 = Subtract(x=w239, y=w237) -> (x-y=w234:dbl)
        n75 = Unbundle By Name(w236) -> ("load"=w235:dbl)
        n76 = Add(x=w235, y=w234) -> (x+y=w233:dbl)
        n77 = call "Convert Data To API String Arguments.vim"("error in (no error)"=w240, "data"=w233) -> ("error out"=w243:errorcluster, "String"=w247:string)  [unwired: 6 in]
        n78 = call-poly <userlib>:"Build Message with Arguments++.vi"("State with Arguments"="API: show", "Arguments (\"\")"=w247, "Target Module (\"\")"="Main" ("Target Module (\"\")")) -> ("State with Arguments out"=w245:string)  [unwired: 12 in]
        n79 = call <vilib>:"Add State(s) to Queue__JKI_lib_State_Machine.vi"("State(s) in Front (\"\")"=w245, "State(s) in (\"\")"=w249) -> ("States Out"=w250:string)  [unwired: 13 in]
      }
      frame "API: TAP" {
        # "#CSM \"Category Seperator\"\nDo not put any code in this frame."
        n80 = call "Convert API String Arguments to Data.vim"("Type"=0, "error in (no error)"=w263, "String"=w265) -> ("error"=w257:errorcluster, "Data"=w262:i32)  [unwired: 5 in]
        n81 = Unbundle By Name(w261) -> ("timeseq.SEQ"=w251:i32[], "TAPSEQ"=w252:i32[], "load"=w254:dbl)
        n82 = Build Array (concatenate)(w252, w262) -> (w259:i32[])
        n83 = Array Size(array=w251) -> (size(s)=w258:i32)
        n84 = Array Size(array=w259) -> (size(s)=w271:i32)
        n85 = Equal?(x=w251, y=w259) -> (x = y?=w272:bool[])
        n86 = Equal?(x=w258, y=w271) -> (x = y?=w269:bool)
        n87 = And Array Elements(Boolean array=w272) -> (logical AND=w270:bool)
        n88 = case shown="True" w270 {
          tunnel: w269 -> [_ w284]
          tunnel: [w277 w283] -> w266
          tunnel: [-1 ("TMO") w282] -> w256
          tunnel: [0.0 ("load") w281] -> w255
          tunnel: w254 -> [_ w280]
          tunnel: [i32[] [] ("timeseq.SEQ") w279] -> w253
          tunnel: w251 -> [_ w279]
          frame False {
            n89 = call-poly <userlib>:"Build Message with Arguments++.vi"("State with Arguments"="API: OVER", "Target Module (\"\")"="Main" ("Target Module (\"\")")) -> ("State with Arguments out"=w277:string)  [unwired: 13 in]
          }
          frame True {
            n90 = case shown="True" w284 {
              tunnel: ["" ("State with Arguments out") w290] -> w283
              tunnel: [100 ("TMO") -1 ("TMO")] -> w282
              tunnel: [w285 0.0] -> w281
              tunnel: w280 -> [w285 _]
              frame False {
              }
              frame True {
                w291 = "Main" ("Target Module (\"\")")
                n91 = call-poly <userlib>:"Build Message with Arguments++.vi"("State with Arguments"="API: PASS", "Arguments (\"\")"=w291, "Target Module (\"\")"=w291) -> ("State with Arguments out"=w290:string)  [unwired: 12 in]
              }
            }
          }
        }
        n92 = Bundle By Name(cluster=w261, "TAPSEQ"=w259, "load"=w255, "timeseq.SEQ"=w253) -> (w260:T5)
        n93 = call <vilib>:"Add State(s) to Queue__JKI_lib_State_Machine.vi"("State(s) in Front (\"\")"=w266, "State(s) in (\"\")"=w267) -> ("States Out"=w268:string)  [unwired: 13 in]
      }
      frame "---------- Action ----------" {
        # "#CSM \"Category Seperator\"\nDo not put any code in this frame."
        n94 = call <vilib>:"Add State(s) to Queue__JKI_lib_State_Machine.vi"("State(s) in (\"\")"=w296) -> ("States Out"=w295:string)  [unwired: 14 in]
      }
      frame "Action: SEQ" {
        # "#CSM API Example\nCopy/Rename this case for your own API"
        n95 = Unbundle By Name(w311) -> ("timeseq.SEQ"=w299:i32[])
        n96 = call-poly <vilib>:"Random Number (Range).vi"("lower bound (0)"=u64 1, "upper bound (100)"=u64 4) -> ("number"=w309:u64)  [unwired: 9 in]
        n97 = Build Array (concatenate)(w299, w309) -> (w310:u64[])
        n98 = Array Size(array=w299) -> (size(s)=w300:i32)
        n99 = Bundle By Name(cluster=w311, "timeseq.SEQ"=w310, "score"=w300) -> (w312:T5)
        n100 = call "Convert Data To API String Arguments.vim"("error in (no error)"=w298, "data"=w310) -> ("error out"=w313:errorcluster, "String"=w303:string)  [unwired: 6 in]
        n101 = call-poly <userlib>:"Build Message with Arguments++.vi"("State with Arguments"="API: BLINK", "Arguments (\"\")"=w303, "Target Module (\"\")"="Main" ("Target Module (\"\")")) -> ("State with Arguments out"=w301:string)  [unwired: 12 in]
        n102 = call <vilib>:"Add State(s) to Queue__JKI_lib_State_Machine.vi"("State(s) in Front (\"\")"=w301, "State(s) in (\"\")"=w305) -> ("States Out"=w306:string)  [unwired: 13 in]
      }
      frame "Action: CNT" {
        # "#CSM API Example\nCopy/Rename this case for your own API"
        n103 = Unbundle By Name(w322) -> ("load"=w317:dbl, "current"=w327:timestamp, "timeseq.time"=w326:i32, "timeseq.SEQ"=w314:i32[])
        n104 = Get Date/Time In Seconds() -> (seconds since 1Jan1904=w328:timestamp)
        n105 = Subtract(x=w328, y=w327) -> (x-y=w316:dbl)
        n106 = Add(x=w317, y=w316) -> (x+y=w318:dbl)
        n107 = call "Convert Data To API String Arguments.vim"("error in (no error)"=w320, "data"=w318) -> ("error out"=w319:errorcluster, "String"=w331:string)  [unwired: 6 in]
        n108 = Greater?(x=w318, y=w326) -> (0:w325:bool)
        n109 = case shown="True" w325 {
          tunnel: ["" ("State with Arguments out") w340] -> w324
          tunnel: [100 -1] -> w323
          tunnel: [w335 i32[] [] ("timeseq.SEQ")] -> w315
          tunnel: w314 -> [w335 _]
          frame False {
          }
          frame True {
            n110 = call-poly <userlib>:"Build Message with Arguments++.vi"("State with Arguments"="API: OVER", "Target Module (\"\")"="Main" ("Target Module (\"\")")) -> ("State with Arguments out"=w340:string)  [unwired: 13 in]
          }
        }
        n111 = Bundle By Name(cluster=w322, "elapsed"=w316, "timeseq.SEQ"=w315) -> (w321:T5)
        n112 = call-poly <userlib>:"Build Message with Arguments++.vi"("State with Arguments"="API: show", "Arguments (\"\")"=w331, "Target Module (\"\")"="Main" ("Target Module (\"\")")) -> ("State with Arguments out"=w329:string)  [unwired: 12 in]
        n113 = call <vilib>:"Add State(s) to Queue__JKI_lib_State_Machine.vi"("State(s) in Front (\"\")"=w329, "State(s) in (\"\")"=w333, "State(s) at Back (\"\")"=w324) -> ("States Out"=w334:string)  [unwired: 12 in]
      }
      frame "Action: EXIT" {
        # "#CSM \"Internal State\"\nThis category is used for holding internal states"
        n114 = Bundle By Name(cluster=w345, "timeseq.SEQ"=i32[] [] ("TAPSEQ")) -> (w344:T5)
        n115 = call <vilib>:"Add State(s) to Queue__JKI_lib_State_Machine.vi"("State(s) in (\"\")"=w348) -> ("States Out"=w347:string)  [unwired: 14 in]
      }
    }
  }
